vi "归一化值设置.vi"(6 "归一化":string, 7 "channel":i32=1 min=1 max=4 step=1, 8 "错误输入（无错误）":errorcluster, 9 "amplifier":i32, 10 "BKNexusD.IPort输入":refnum<k7>) -> (0 "错误输出":errorcluster, 2 "BKNexusD.IPort输出":refnum<k7>, 3 "channel settings":T1)   [LabVIEW 2015]
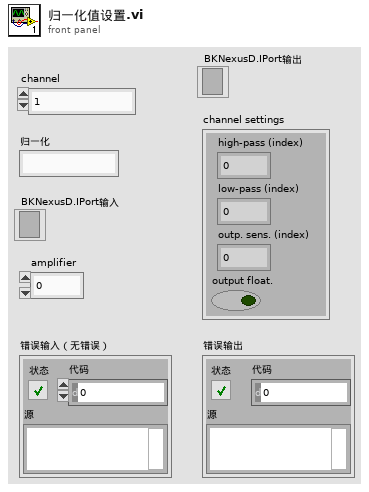
[diagram p1: front panel]
types:
  T1 = cluster{"high-pass (index)":u16, "low-pass (index)":u16, "outp. sens. (index)":u16, "output float.":bool}
  T2 = cluster{"low-pass range":string[], "outp. sens. range":string[], "high-pass range":string[]}
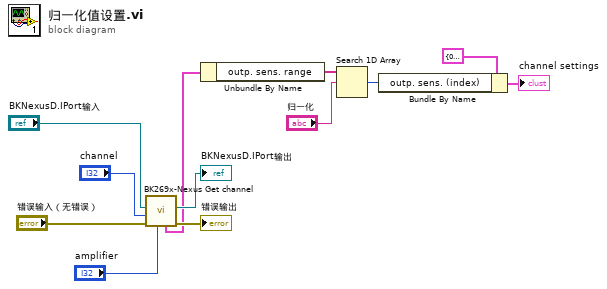
[diagram p0: block diagram]
diagram:
  n1 = call <instrlib>:"BK269x-Nexus Get channel.vi"("amplifier"="amplifier", "error in"="错误输入（无错误）", "channel"="channel", "BKNexusD.IPort"="BKNexusD.IPort输入") -> ("error out"=→"错误输出":errorcluster, "BKNexusD.IPort"=→"BKNexusD.IPort输出":refnum<k7>, "channel settings ranges"=w6:T2)  [unwired: 2 in, 3 out]
  n2 = Unbundle By Name(w6) -> ("outp. sens. range"=w8:string[])
  n3 = Search 1D Array(1D array=w8, element="归一化") -> (index of element=w10:i32)  [unwired: 1 in]
  n4 = Bundle By Name(cluster=T1 {"high-pass (index)"=0, "low-pass (index)"=6, "outp. sens. (index)"=4, "output float."=FALSE} ("channel settings"), "outp. sens. (index)"=w10) -> (→"channel settings":T1)
